vi "Drive Modifications.vi"(1 "Drive Info In":T1) -> (0 "Drive Info Out":T1)   [LabVIEW 2013]
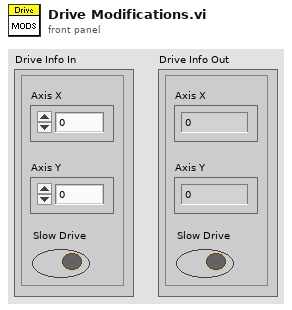
[diagram p1: front panel]
types:
  T1 = cluster{"Axis X":dbl, "Axis Y":dbl, "Slow Drive":bool}
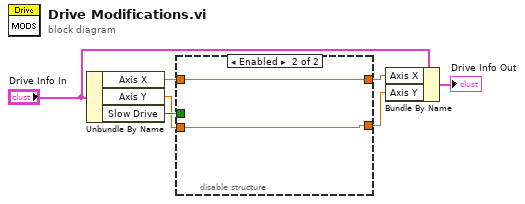
[diagram p0: block diagram]
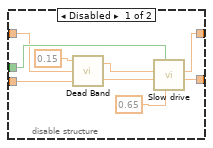
[diagram p2: hidden frame]
diagram:
  n1 = Unbundle By Name("Drive Info In") -> ("Axis X"=w2:dbl, "Axis Y"=w1:dbl, "Slow Drive"=w7:bool)
  n2 = disable-structure shown="Enabled" {
    disable-tunnel: w7 -> [w16 _]
    disable-tunnel: [w14 w18] -> w4
    disable-tunnel: [w13 w17] -> w3
    disable-tunnel: w2 -> [w9 w18]
    disable-tunnel: w1 -> [w8 w17]
    frame Disabled {
      n3 = call "Dead Band.vi"("Axis 2 In"=w8, "Axis 1 In"=w9, "Dead Band"=0.15) -> ("Axis 2 Out"=w11:dbl, "Axis 1 Out"=w12:dbl)
      n4 = call "Slow drive.vi"("Slow drive to"=0.65, "Slow?"=w16, "Y-Axis"=w11, "X-Axis"=w12) -> ("Y - Axis out"=w13:dbl, "X-Axis out"=w14:dbl)  [unwired: 6 in]
    }
    frame Enabled {
    }
  }
  n5 = Bundle By Name(cluster="Drive Info In", "Axis X"=w4, "Axis Y"=w3) -> (→"Drive Info Out":T1)
